vi "Create Font Object.vi"(8 "Error In":errorcluster, 9 "Style":T1, 10 "Size":sgl, 11 "Name":string) -> (0 "Error Out":errorcluster, 3 "Font Object":refnum<k24>)   [LabVIEW 2020, in "Dot Net UI Controls.lvlib"]
uses:
  Dot Net UI Controls.lvlib
  System.Drawing
  Font Style.ctl
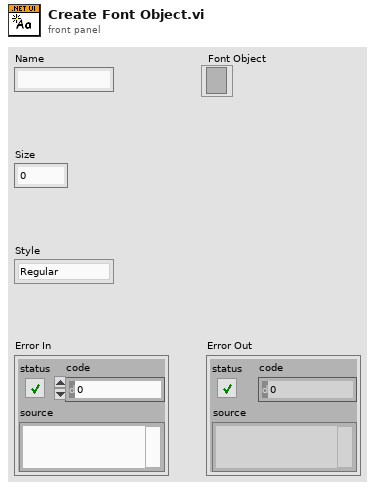
[diagram p1: front panel]
types:
  T1 = typedef "Dot Net UI Controls.lvlib/Font Style.ctl" = enum16{"Regular", "Bold", "Italic", "Underline", "Strikeout"}
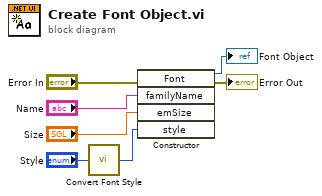
[diagram p0: block diagram]
diagram:
  n1 = call "Convert Font Style.vi"("Font Style In"="Style") -> ("Font Style Out"=w3:i32)
  n2 = constructor class="Font"(error in="Error In", "familyName"="Name", "emSize"="Size", "style"=w3) -> (reference out=→"Font Object":refnum<k24>, error out=→"Error Out":errorcluster)  [unwired: 2 in, 4 out]
